vi "major pro.vi"() -> ()   [LabVIEW 2018]
panel:
  out "tank elert":bool
  out "STATUS":string
  in  "SELECT MODE":T1(ring)
  out "dry":bool
  out "rinse":bool
  out "soak":bool
  in  "?":bool
  out "TIMER":dbl
  out "Tank":dbl(slide) scale=0.0..100.0
  in  "?":bool
  out "Slide":u8(slide) scale=0.0..100.0
  out "wash":bool
  in  "OK Button":bool
  # "Sec"
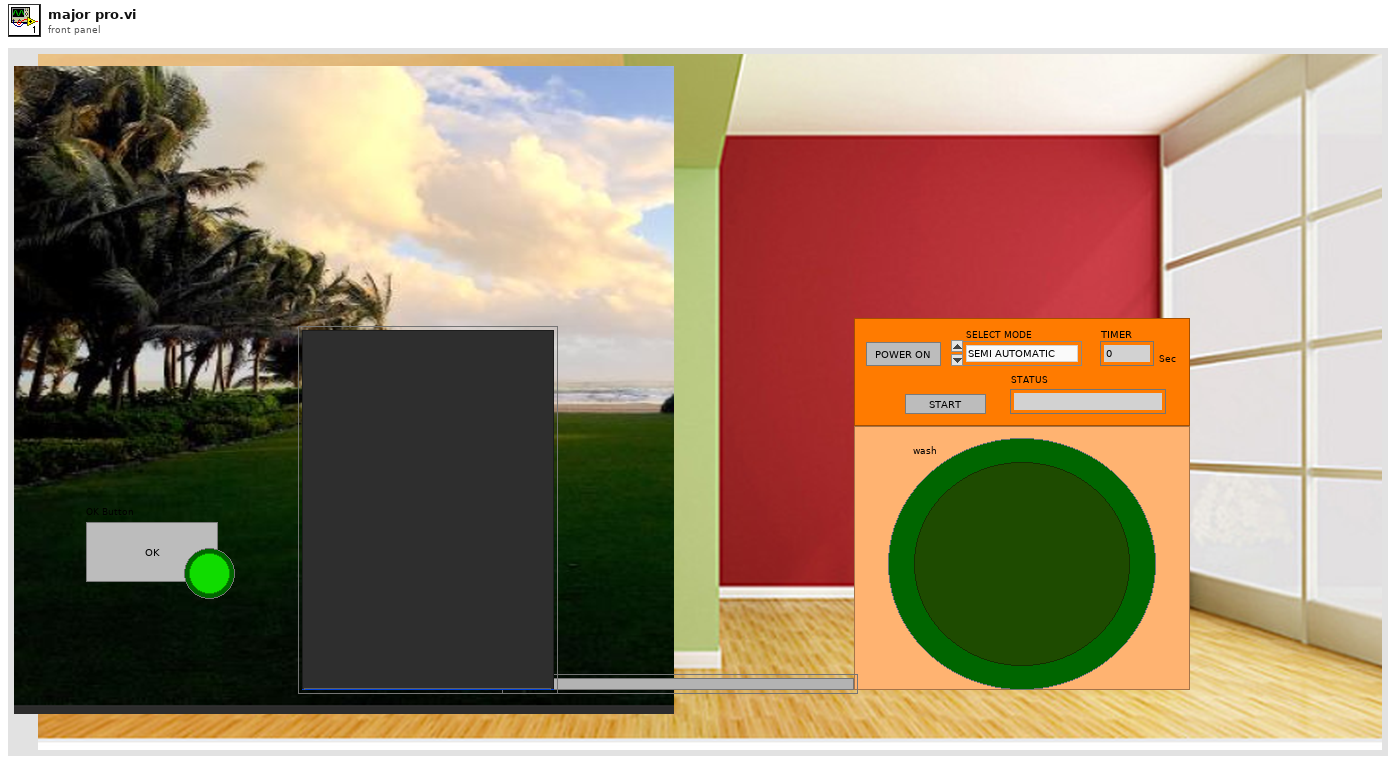
[diagram p1: front panel]
types:
  T1 = enum16{"SEMI AUTOMATIC", "FULLY AUTOMATIC", "RINSING", "DRYING", "SOAKING", "WASHING"}
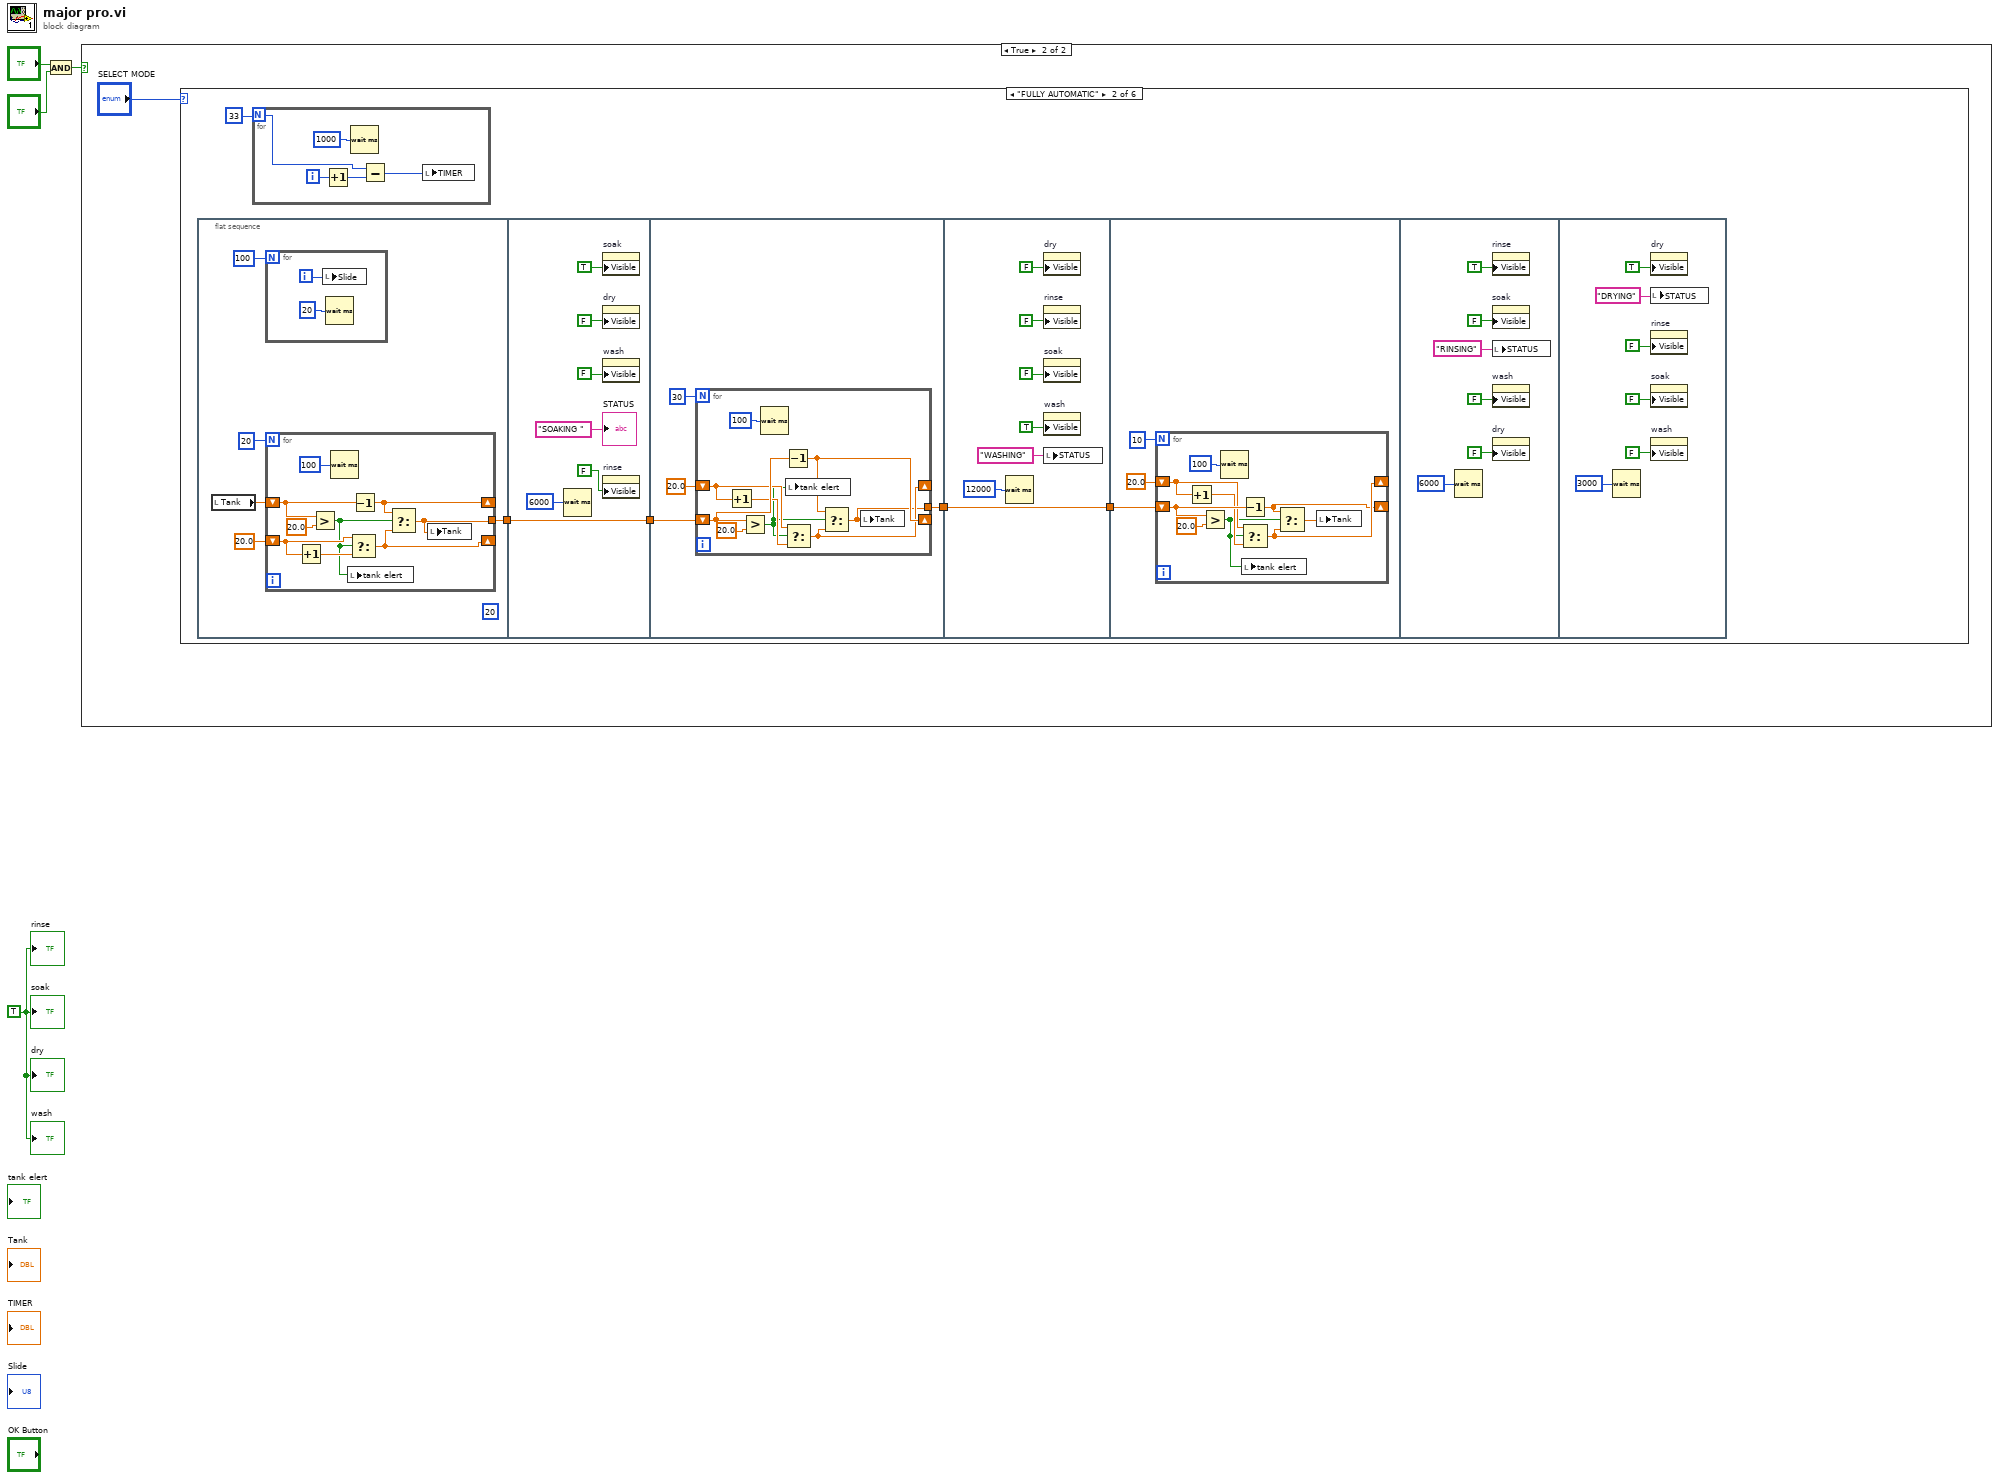
[diagram p0: block diagram]
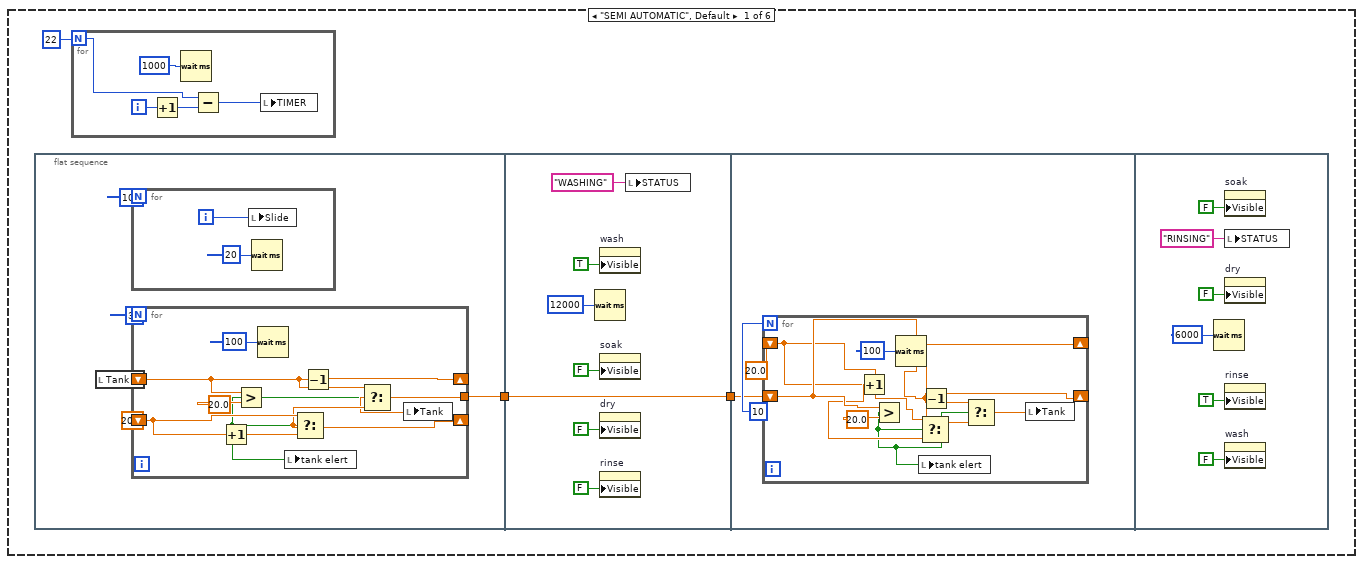
[diagram p3: hidden frame]
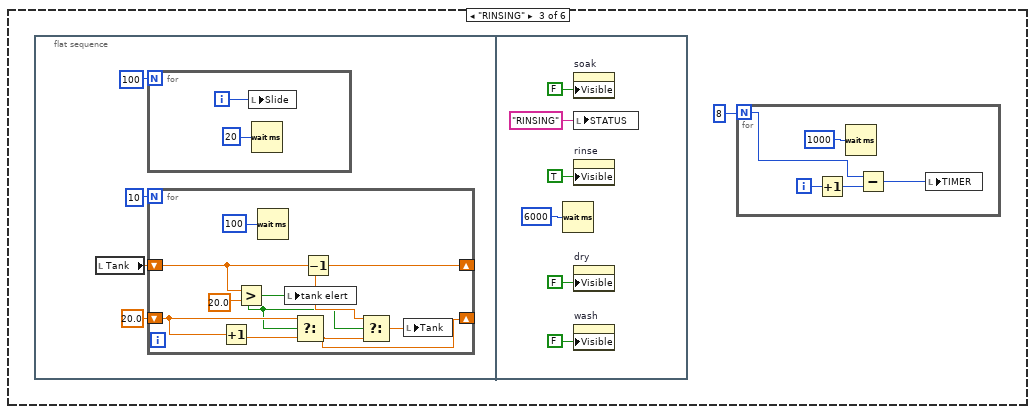
[diagram p4: hidden frame]
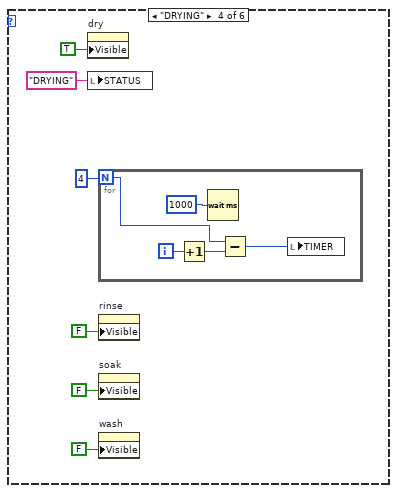
[diagram p5: hidden frame]
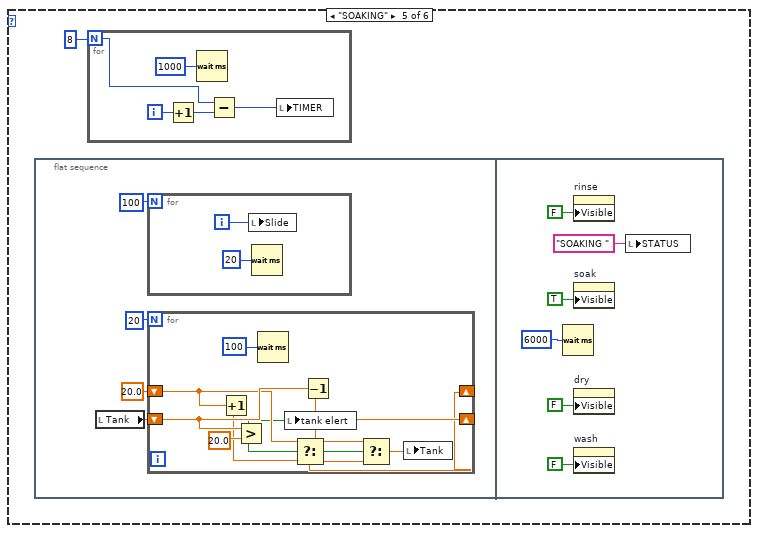
[diagram p6: hidden frame]
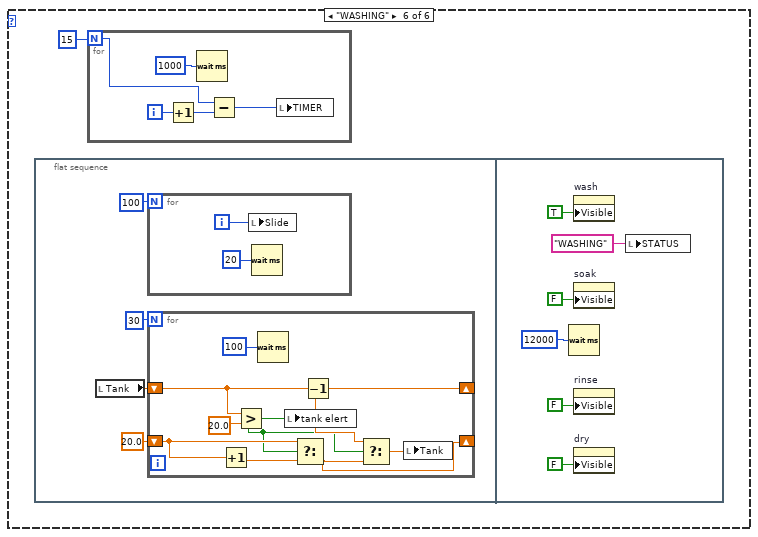
[diagram p7: hidden frame]
diagram:
  w4 = TRUE
  n1 = And(x="?", y="?") -> (x .and. y?=w3:bool)
  n2 = case shown="True" w3 {
    frame False {
    }
    frame True {
      n3 = case shown="\"FULLY AUTOMATIC\"" "SELECT MODE" {
        frame "SEMI AUTOMATIC", Default {
          n4 = flat-sequence {
            tunnel: [w14] -> w7
            tunnel: [w30] -> w8
            tunnel: w7 -> [w30]
            tunnel: w8 -> [w38]
            frame #0 {
              n5 = local read "Tank"() -> (w18:dbl)
              n6 = for {
                N: 100 -> [_]
                i -> [w19]
                n7 = local write "Slide"(w19) -> ()
                n8 = Wait (ms)(milliseconds to wait=u32 20) -> ()  [unwired: 1 out]
              }
              n9 = for {
                N: 30 -> [_]
                shift-right: [w24] -> _
                shift-left: w18 -> [w27]
                shift-right: [w23] -> _
                shift-left: 20.0 ("y") -> [w25]
                tunnel: [w22] -> w14
                n10 = Increment(x=w25) -> (x+1=w26:dbl)
                n11 = Greater?(x=w27, y=20.0) -> (0:w21:bool)
                n12 = Wait (ms)(milliseconds to wait=u32 100) -> ()  [unwired: 1 out]
                n13 = local write "tank elert"(w21) -> ()
                n14 = Select(t=w25, s=w21, f=w26) -> (s? t:f=w23:dbl)
                n15 = Decrement(x=w27) -> (x-1=w24:dbl)
                n16 = Select(t=w24, s=w21, f=w23) -> (s? t:f=w22:dbl)
                n17 = local write "Tank"(w22) -> ()
              }
            }
            frame #1 {
              n18 = Wait (ms)(milliseconds to wait=u32 12000) -> ()  [unwired: 1 out]
              n19 = property on="wash" class="Bool (strict)"("Visible"=TRUE) -> ()  [unwired: 2 in, 2 out]
              n20 = property on="soak" class="Bool (strict)"("Visible"=FALSE) -> ()  [unwired: 2 in, 2 out]
              n21 = property on="dry" class="Bool (strict)"("Visible"=FALSE) -> ()  [unwired: 2 in, 2 out]
              n22 = property on="rinse" class="Bool (strict)"("Visible"=FALSE) -> ()  [unwired: 2 in, 2 out]
              n23 = local write "STATUS"("WASHING" ("STATUS")) -> ()
            }
            frame #2 {
              n24 = for {
                N: 10 -> [_]
                shift-right: [w42] -> _
                shift-left: w38 -> [w46]
                shift-right: [w41] -> _
                shift-left: 20.0 ("y") -> [w43]
                n25 = Increment(x=w43) -> (x+1=w44:dbl)
                n26 = Greater?(x=w46, y=20.0) -> (0:w40:bool)
                n27 = Wait (ms)(milliseconds to wait=u32 100) -> ()  [unwired: 1 out]
                n28 = local write "tank elert"(w40) -> ()
                n29 = Select(t=w43, s=w40, f=w44) -> (s? t:f=w41:dbl)
                n30 = Decrement(x=w46) -> (x-1=w42:dbl)
                n31 = Select(t=w42, s=w40, f=w41) -> (s? t:f=w45:dbl)
                n32 = local write "Tank"(w45) -> ()
              }
            }
            frame #3 {
              n33 = Wait (ms)(milliseconds to wait=u32 6000) -> ()  [unwired: 1 out]
              n34 = property on="soak" class="Bool (strict)"("Visible"=FALSE) -> ()  [unwired: 2 in, 2 out]
              n35 = local write "STATUS"("RINSING" ("STATUS")) -> ()
              n36 = property on="dry" class="Bool (strict)"("Visible"=FALSE) -> ()  [unwired: 2 in, 2 out]
              n37 = property on="rinse" class="Bool (strict)"("Visible"=TRUE) -> ()  [unwired: 2 in, 2 out]
              n38 = property on="wash" class="Bool (strict)"("Visible"=FALSE) -> ()  [unwired: 2 in, 2 out]
            }
          }
          n39 = for {
            N: 22 -> [w13]
            i -> [w12]
            n40 = Increment(x=w12) -> (x+1=w10:i32)
            n41 = Wait (ms)(milliseconds to wait=u32 1000) -> ()  [unwired: 1 out]
            n42 = Subtract(x=w13, y=w10) -> (x-y=w11:i32)
            n43 = local write "TIMER"(w11) -> ()
          }
        }
        frame "FULLY AUTOMATIC" {
          n44 = flat-sequence {
            tunnel: [w65] -> w55
            tunnel: [w81] -> w58
            tunnel: w55 -> [w81]
            tunnel: w58 -> [w89]
            tunnel: [w88] -> w56
            tunnel: [w101] -> w59
            tunnel: w56 -> [w101]
            tunnel: w59 -> [w110]
            frame #0 {
              (unwired) 20
              n45 = local read "Tank"() -> (w67:dbl)
              n46 = for {
                N: 100 -> [_]
                i -> [w79]
                n47 = local write "Slide"(w79) -> ()
                n48 = Wait (ms)(milliseconds to wait=u32 20) -> ()  [unwired: 1 out]
              }
              n49 = for {
                N: 20 -> [_]
                shift-right: [w73] -> _
                shift-left: w67 -> [w76]
                shift-right: [w72] -> _
                shift-left: 20.0 ("y") -> [w74]
                tunnel: [w71] -> w65
                n50 = Increment(x=w74) -> (x+1=w75:dbl)
                n51 = Greater?(x=w76, y=20.0) -> (0:w70:bool)
                n52 = Wait (ms)(milliseconds to wait=u32 100) -> ()  [unwired: 1 out]
                n53 = local write "tank elert"(w70) -> ()
                n54 = Select(t=w74, s=w70, f=w75) -> (s? t:f=w72:dbl)
                n55 = Decrement(x=w76) -> (x-1=w73:dbl)
                n56 = Select(t=w73, s=w70, f=w72) -> (s? t:f=w71:dbl)
                n57 = local write "Tank"(w71) -> ()
              }
            }
            frame #1 {
              n58 = Wait (ms)(milliseconds to wait=u32 6000) -> ()  [unwired: 1 out]
              n59 = property on="soak" class="Bool (strict)"("Visible"=TRUE) -> ()  [unwired: 2 in, 2 out]
              n60 = property on="dry" class="Bool (strict)"("Visible"=FALSE) -> ()  [unwired: 2 in, 2 out]
              n61 = property on="wash" class="Bool (strict)"("Visible"=FALSE) -> ()  [unwired: 2 in, 2 out]
              n62 = property on="rinse" class="Bool (strict)"("Visible"=FALSE) -> ()  [unwired: 2 in, 2 out]
              "STATUS" <- "SOAKING " ("STATUS")
            }
            frame #2 {
              n63 = for {
                N: 30 -> [_]
                shift-right: [w95] -> _
                shift-left: w89 -> [w98]
                shift-right: [w94] -> _
                shift-left: 20.0 ("y") -> [w96]
                tunnel: [w93] -> w88
                n64 = Increment(x=w96) -> (x+1=w97:dbl)
                n65 = Greater?(x=w98, y=20.0) -> (0:w92:bool)
                n66 = Wait (ms)(milliseconds to wait=u32 100) -> ()  [unwired: 1 out]
                n67 = Decrement(x=w98) -> (x-1=w95:dbl)
                n68 = Select(t=w96, s=w92, f=w97) -> (s? t:f=w94:dbl)
                n69 = local write "tank elert"(w92) -> ()
                n70 = Select(t=w95, s=w92, f=w94) -> (s? t:f=w93:dbl)
                n71 = local write "Tank"(w93) -> ()
              }
            }
            frame #3 {
              n72 = Wait (ms)(milliseconds to wait=u32 12000) -> ()  [unwired: 1 out]
              n73 = property on="dry" class="Bool (strict)"("Visible"=FALSE) -> ()  [unwired: 2 in, 2 out]
              n74 = property on="rinse" class="Bool (strict)"("Visible"=FALSE) -> ()  [unwired: 2 in, 2 out]
              n75 = property on="soak" class="Bool (strict)"("Visible"=FALSE) -> ()  [unwired: 2 in, 2 out]
              n76 = property on="wash" class="Bool (strict)"("Visible"=TRUE) -> ()  [unwired: 2 in, 2 out]
              n77 = local write "STATUS"("WASHING" ("STATUS")) -> ()
            }
            frame #4 {
              n78 = for {
                N: 10 -> [_]
                shift-right: [w112] -> _
                shift-left: w110 -> [w117]
                shift-right: [w113] -> _
                shift-left: 20.0 ("y") -> [w114]
                n79 = Increment(x=w114) -> (x+1=w115:dbl)
                n80 = Greater?(x=w117, y=20.0) -> (0:w111:bool)
                n81 = Wait (ms)(milliseconds to wait=u32 100) -> ()  [unwired: 1 out]
                n82 = Decrement(x=w117) -> (x-1=w112:dbl)
                n83 = Select(t=w114, s=w111, f=w115) -> (s? t:f=w113:dbl)
                n84 = local write "tank elert"(w111) -> ()
                n85 = Select(t=w112, s=w111, f=w113) -> (s? t:f=w116:dbl)
                n86 = local write "Tank"(w116) -> ()
              }
            }
            frame #5 {
              n87 = Wait (ms)(milliseconds to wait=u32 6000) -> ()  [unwired: 1 out]
              n88 = property on="rinse" class="Bool (strict)"("Visible"=TRUE) -> ()  [unwired: 2 in, 2 out]
              n89 = property on="soak" class="Bool (strict)"("Visible"=FALSE) -> ()  [unwired: 2 in, 2 out]
              n90 = local write "STATUS"("RINSING" ("STATUS")) -> ()
              n91 = property on="wash" class="Bool (strict)"("Visible"=FALSE) -> ()  [unwired: 2 in, 2 out]
              n92 = property on="dry" class="Bool (strict)"("Visible"=FALSE) -> ()  [unwired: 2 in, 2 out]
            }
            frame #6 {
              n93 = Wait (ms)(milliseconds to wait=u32 3000) -> ()  [unwired: 1 out]
              n94 = property on="dry" class="Bool (strict)"("Visible"=TRUE) -> ()  [unwired: 2 in, 2 out]
              n95 = local write "STATUS"("DRYING" ("STATUS")) -> ()
              n96 = property on="rinse" class="Bool (strict)"("Visible"=FALSE) -> ()  [unwired: 2 in, 2 out]
              n97 = property on="soak" class="Bool (strict)"("Visible"=FALSE) -> ()  [unwired: 2 in, 2 out]
              n98 = property on="wash" class="Bool (strict)"("Visible"=FALSE) -> ()  [unwired: 2 in, 2 out]
            }
          }
          n99 = for {
            N: 33 -> [w64]
            i -> [w63]
            n100 = Increment(x=w63) -> (x+1=w62:i32)
            n101 = Wait (ms)(milliseconds to wait=u32 1000) -> ()  [unwired: 1 out]
            n102 = Subtract(x=w64, y=w62) -> (x-y=w60:i32)
            n103 = local write "TIMER"(w60) -> ()
          }
        }
        frame "RINSING" {
          n104 = flat-sequence {
            frame #0 {
              n105 = local read "Tank"() -> (w139:dbl)
              n106 = for {
                N: 100 -> [_]
                i -> [w142]
                n107 = local write "Slide"(w142) -> ()
                n108 = Wait (ms)(milliseconds to wait=u32 20) -> ()  [unwired: 1 out]
              }
              n109 = for {
                N: 10 -> [_]
                shift-right: [w146] -> _
                shift-left: w139 -> [w150]
                shift-right: [w145] -> _
                shift-left: 20.0 ("y") -> [w147]
                n110 = Increment(x=w147) -> (x+1=w148:dbl)
                n111 = Greater?(x=w150, y=20.0) -> (0:w144:bool)
                n112 = Wait (ms)(milliseconds to wait=u32 100) -> ()  [unwired: 1 out]
                n113 = local write "tank elert"(w144) -> ()
                n114 = Select(t=w147, s=w144, f=w148) -> (s? t:f=w145:dbl)
                n115 = Decrement(x=w150) -> (x-1=w146:dbl)
                n116 = Select(t=w146, s=w144, f=w145) -> (s? t:f=w149:dbl)
                n117 = local write "Tank"(w149) -> ()
              }
            }
            frame #1 {
              n118 = Wait (ms)(milliseconds to wait=u32 6000) -> ()  [unwired: 1 out]
              n119 = property on="soak" class="Bool (strict)"("Visible"=FALSE) -> ()  [unwired: 2 in, 2 out]
              n120 = local write "STATUS"("RINSING" ("STATUS")) -> ()
              n121 = property on="rinse" class="Bool (strict)"("Visible"=TRUE) -> ()  [unwired: 2 in, 2 out]
              n122 = property on="dry" class="Bool (strict)"("Visible"=FALSE) -> ()  [unwired: 2 in, 2 out]
              n123 = property on="wash" class="Bool (strict)"("Visible"=FALSE) -> ()  [unwired: 2 in, 2 out]
            }
          }
          n124 = for {
            N: 8 -> [w137]
            i -> [w136]
            n125 = Increment(x=w136) -> (x+1=w135:i32)
            n126 = Wait (ms)(milliseconds to wait=u32 1000) -> ()  [unwired: 1 out]
            n127 = Subtract(x=w137, y=w135) -> (x-y=w134:i32)
            n128 = local write "TIMER"(w134) -> ()
          }
        }
        frame "DRYING" {
          n129 = property on="dry" class="Bool (strict)"("Visible"=TRUE) -> ()  [unwired: 2 in, 2 out]
          n130 = local write "STATUS"("DRYING" ("STATUS")) -> ()
          n131 = for {
            N: 4 -> [w168]
            i -> [w167]
            n132 = Increment(x=w167) -> (x+1=w165:i32)
            n133 = Wait (ms)(milliseconds to wait=u32 1000) -> ()  [unwired: 1 out]
            n134 = Subtract(x=w168, y=w165) -> (x-y=w166:i32)
            n135 = local write "TIMER"(w166) -> ()
          }
          n136 = property on="rinse" class="Bool (strict)"("Visible"=FALSE) -> ()  [unwired: 2 in, 2 out]
          n137 = property on="soak" class="Bool (strict)"("Visible"=FALSE) -> ()  [unwired: 2 in, 2 out]
          n138 = property on="wash" class="Bool (strict)"("Visible"=FALSE) -> ()  [unwired: 2 in, 2 out]
        }
        frame "SOAKING" {
          n139 = flat-sequence {
            frame #0 {
              n140 = local read "Tank"() -> (w179:dbl)
              n141 = for {
                N: 100 -> [_]
                i -> [w180]
                n142 = local write "Slide"(w180) -> ()
                n143 = Wait (ms)(milliseconds to wait=u32 20) -> ()  [unwired: 1 out]
              }
              n144 = for {
                N: 20 -> [_]
                shift-right: [w184] -> _
                shift-left: w179 -> [w188]
                shift-right: [w183] -> _
                shift-left: 20.0 ("y") -> [w185]
                n145 = Increment(x=w185) -> (x+1=w186:dbl)
                n146 = Greater?(x=w188, y=20.0) -> (0:w182:bool)
                n147 = Wait (ms)(milliseconds to wait=u32 100) -> ()  [unwired: 1 out]
                n148 = local write "tank elert"(w182) -> ()
                n149 = Select(t=w185, s=w182, f=w186) -> (s? t:f=w183:dbl)
                n150 = Decrement(x=w188) -> (x-1=w184:dbl)
                n151 = Select(t=w184, s=w182, f=w183) -> (s? t:f=w187:dbl)
                n152 = local write "Tank"(w187) -> ()
              }
            }
            frame #1 {
              n153 = Wait (ms)(milliseconds to wait=u32 6000) -> ()  [unwired: 1 out]
              n154 = property on="rinse" class="Bool (strict)"("Visible"=FALSE) -> ()  [unwired: 2 in, 2 out]
              n155 = property on="soak" class="Bool (strict)"("Visible"=TRUE) -> ()  [unwired: 2 in, 2 out]
              n156 = property on="dry" class="Bool (strict)"("Visible"=FALSE) -> ()  [unwired: 2 in, 2 out]
              n157 = property on="wash" class="Bool (strict)"("Visible"=FALSE) -> ()  [unwired: 2 in, 2 out]
              n158 = local write "STATUS"("SOAKING " ("STATUS")) -> ()
            }
          }
          n159 = for {
            N: 8 -> [w174]
            i -> [w173]
            n160 = Increment(x=w173) -> (x+1=w171:i32)
            n161 = Wait (ms)(milliseconds to wait=u32 1000) -> ()  [unwired: 1 out]
            n162 = Subtract(x=w174, y=w171) -> (x-y=w172:i32)
            n163 = local write "TIMER"(w172) -> ()
          }
        }
        frame "WASHING" {
          n164 = flat-sequence {
            frame #0 {
              n165 = local read "Tank"() -> (w204:dbl)
              n166 = for {
                N: 100 -> [_]
                i -> [w207]
                n167 = local write "Slide"(w207) -> ()
                n168 = Wait (ms)(milliseconds to wait=u32 20) -> ()  [unwired: 1 out]
              }
              n169 = for {
                N: 30 -> [_]
                shift-right: [w211] -> _
                shift-left: w204 -> [w215]
                shift-right: [w210] -> _
                shift-left: 20.0 ("y") -> [w212]
                n170 = Increment(x=w212) -> (x+1=w213:dbl)
                n171 = Greater?(x=w215, y=20.0) -> (0:w209:bool)
                n172 = Wait (ms)(milliseconds to wait=u32 100) -> ()  [unwired: 1 out]
                n173 = local write "tank elert"(w209) -> ()
                n174 = Select(t=w212, s=w209, f=w213) -> (s? t:f=w210:dbl)
                n175 = Decrement(x=w215) -> (x-1=w211:dbl)
                n176 = Select(t=w211, s=w209, f=w210) -> (s? t:f=w214:dbl)
                n177 = local write "Tank"(w214) -> ()
              }
            }
            frame #1 {
              n178 = Wait (ms)(milliseconds to wait=u32 12000) -> ()  [unwired: 1 out]
              n179 = property on="wash" class="Bool (strict)"("Visible"=TRUE) -> ()  [unwired: 2 in, 2 out]
              n180 = property on="soak" class="Bool (strict)"("Visible"=FALSE) -> ()  [unwired: 2 in, 2 out]
              n181 = property on="rinse" class="Bool (strict)"("Visible"=FALSE) -> ()  [unwired: 2 in, 2 out]
              n182 = property on="dry" class="Bool (strict)"("Visible"=FALSE) -> ()  [unwired: 2 in, 2 out]
              n183 = local write "STATUS"("WASHING" ("STATUS")) -> ()
            }
          }
          n184 = for {
            N: 15 -> [w201]
            i -> [w200]
            n185 = Increment(x=w200) -> (x+1=w199:i32)
            n186 = Wait (ms)(milliseconds to wait=u32 1000) -> ()  [unwired: 1 out]
            n187 = Subtract(x=w201, y=w199) -> (x-y=w198:i32)
            n188 = local write "TIMER"(w198) -> ()
          }
        }
      }
    }
  }
  "rinse" <- w4
  "soak" <- w4
  "dry" <- w4
  "wash" <- w4
